vi "Modified Data File Current Mode.vi"(7 "Current Mode":u8[][](array[numeric]), 8 "modified error":errorcluster, 9 "modified data":path=path "C:/Users/User/Desktop/test.csv", 10 "original error":errorcluster, 11 "original data":path=path "C:/Users/User/Desktop/test.csv") -> (2 "original error out":errorcluster, 3 "original data out":path)   [LabVIEW 2023]
uses:
  <vilib>/Utility/error.llb/DialogType.ctl
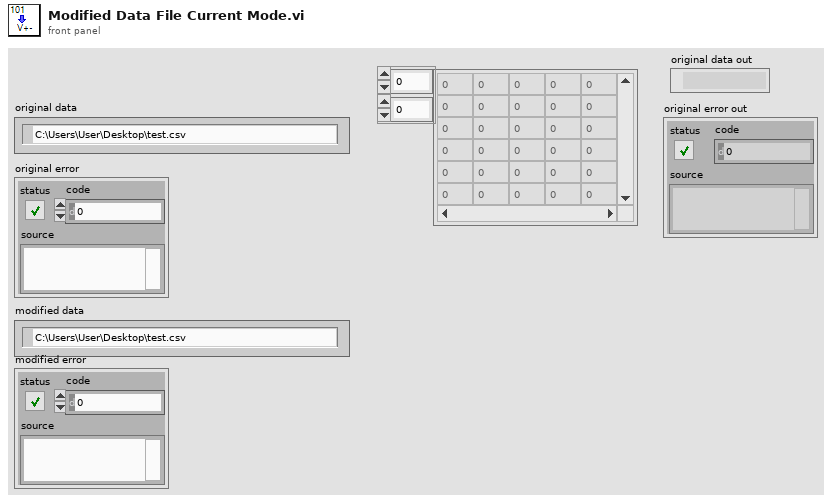
[diagram p1: front panel]
types:
  T1 = enum16{"open", "replace", "create", "open or create", "replace or create", "replace or create with confirmation"}
  T2 = typedef "DialogType.ctl" = u16
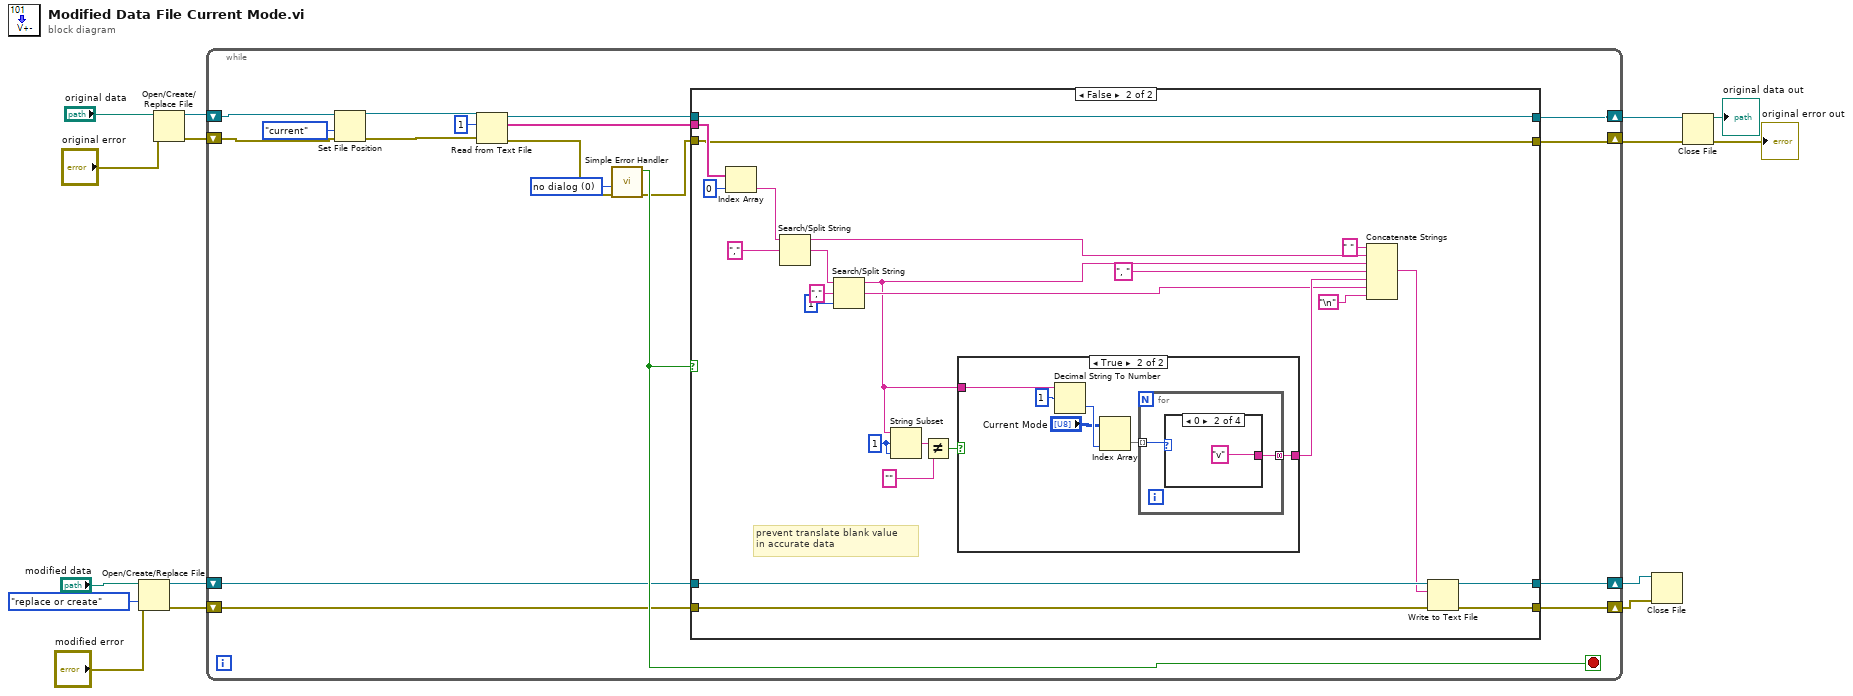
[diagram p0: block diagram]
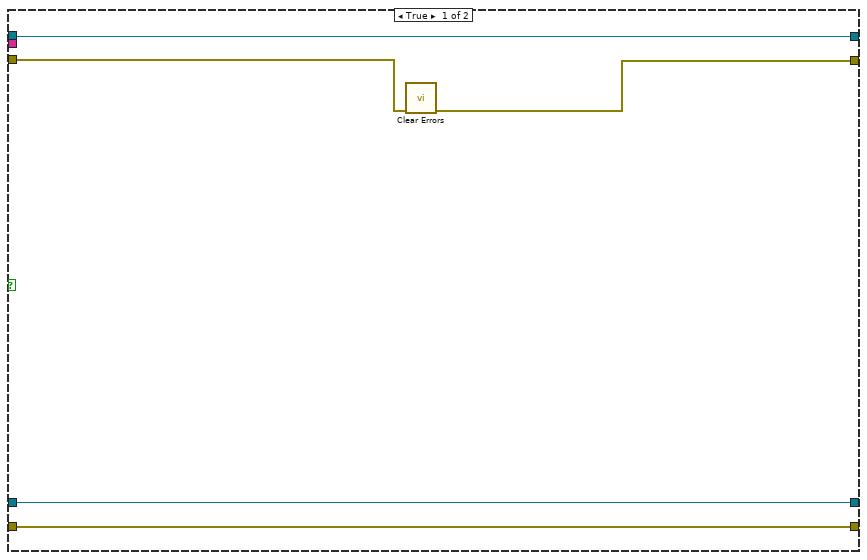
[diagram p2: hidden frame]
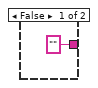
[diagram p3: hidden frame]
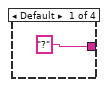
[diagram p4: hidden frame]
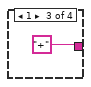
[diagram p5: hidden frame]
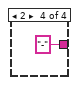
[diagram p6: hidden frame]
diagram:
  n1 = Open/Create/Replace File(file path (use dialog)="modified data", error in="modified error", operation (0:open)=T1."replace or create") -> (refnum out=w10:refnum<file>, error out=w9:errorcluster)  [unwired: 3 in, 1 out]
  n2 = Open/Create/Replace File(file path (use dialog)="original data", error in="original error") -> (refnum out=w12:refnum<file>, error out=w13:errorcluster)  [unwired: 4 in, 1 out]
  n3 = while {
    shift-right: [w25] -> w3
    shift-left: w13 -> [w32]
    shift-right: [w24] -> w14
    shift-left: w12 -> [w23]
    shift-right: [w18] -> w5
    shift-left: w10 -> [w20]
    shift-right: [w17] -> w4
    shift-left: w9 -> [w19]
    stop <- w29 stop-if-true
    w30 = T2 0 items=["no dialog", "OK message", "continue or stop message", "OK message + warnings", "continue/stop + warnings"] ("type of dialog (OK msg:1)")
    n4 = Set File Position(refnum=w23, from (0:start)=enum16{"start", "end", "current"}."current", error in=w32) -> (refnum out=w22:refnum<file>, error out=w21:errorcluster)  [unwired: 1 in]
    n5 = Read from Text File(file (use dialog)=w22, count=1, error in=w21) -> (refnum out=w27:refnum<file>, text=w28:string[], error out=w26:errorcluster)  [unwired: 1 in, 1 out]
    n6 = call <vilib>:"Simple Error Handler.vi"("type of dialog (OK msg:1)"=w30, "error in (no error)"=w26) -> ("error?"=w29:bool, "error out"=w16:errorcluster)  [unwired: 3 in, 3 out]
    n7 = case shown="False" w29 {
      tunnel: w28 -> [_ w56]
      tunnel: w27 -> [w38 w53]
      tunnel: w16 -> [w35 w52]
      tunnel: [w38 w53] -> w24
      tunnel: [w34 w52] -> w25
      tunnel: w20 -> [w37 w51]
      tunnel: w19 -> [w36 w50]
      tunnel: [w37 w49] -> w18
      tunnel: [w36 w48] -> w17
      frame True {
        n8 = call <vilib>:"Clear Errors.vi"("error in (no error)"=w35) -> ("error out"=w34:errorcluster)  [unwired: 5 in, 1 out]
      }
      frame False {
        w42 = 1 ("offset (0)")
        # "prevent translate blank value\nin accurate data"
        n9 = Index Array(array=w56, index=0) -> (element=w54:string)
        n10 = Search/Split String(string=w54, search string/char (-)=",") -> (substring before match=w62:string, match + rest of string=w61:string)  [unwired: 1 in, 1 out]
        n11 = Search/Split String(string=w61, search string/char (-)=",", offset (0)=1) -> (substring before match=w43:string, match + rest of string=w45:string)  [unwired: 1 out]
        n12 = String Subset(string=w43, offset (0)=w42, length (rest)=w42) -> (substring=w41:string)
        n13 = Not Equal?(x=w41, y="") -> (x != y?=w40:bool)
        n14 = case shown="True" w40 {
          tunnel: ["" w70] -> w63
          tunnel: w43 -> [_ w65]
          frame False {
          }
          frame True {
            n15 = Decimal String To Number(string=w65, offset=1) -> (number=w68:i32)  [unwired: 1 in, 1 out]
            n16 = Index Array(array="Current Mode", index (col)=w68) -> (element=w69:u8[])  [unwired: 1 in]
            n17 = for {
              tunnel: w69 -> [w72] mode=indexing
              tunnel: [w71] -> w70 mode=concatenating
              n18 = case shown="0" w72 {
                tunnel: ["?" "v" "+" "-"] -> w71
                frame Default {
                }
                frame 0 {
                }
                frame 1 {
                }
                frame 2 {
                }
              }
            }
          }
        }
        n19 = Concatenate Strings(" " ("string"), w62, w43, ", " ("string"), w63, w45, "\n") -> (w47:string)
        n20 = Write to Text File(file (use dialog)=w51, text=w47, error in=w50) -> (refnum out=w49:refnum<file>, error out=w48:errorcluster)  [unwired: 1 in, 1 out]
      }
    }
  }
  n21 = Close File(refnum=w5, error in=w4) -> ()  [unwired: 2 out]
  n22 = Close File(refnum=w14, error in=w3) -> (path=→"original data out":path, error out=→"original error out":errorcluster)
